vi "writeSVs.vi"(8 "error in (no error)":errorcluster, 11 "LoopTimer in":refnum<class "LoopTimer.lvclass">) -> (0 "error out":errorcluster, 3 "LoopTimer out":refnum<class "LoopTimer.lvclass">)   [LabVIEW 2013, in "ComponentData.lvlib" / "LoopTimer.lvclass"]
uses:
  <userlib>/Common/Component/common_application/RT/ComponentData/LoopTimer/LoopTimer.lvclass
  <userlib>/Common/Component/common_application/RT/ComponentData/LoopTimer/LoopTimer.lvclass/LoopTimer.ctl
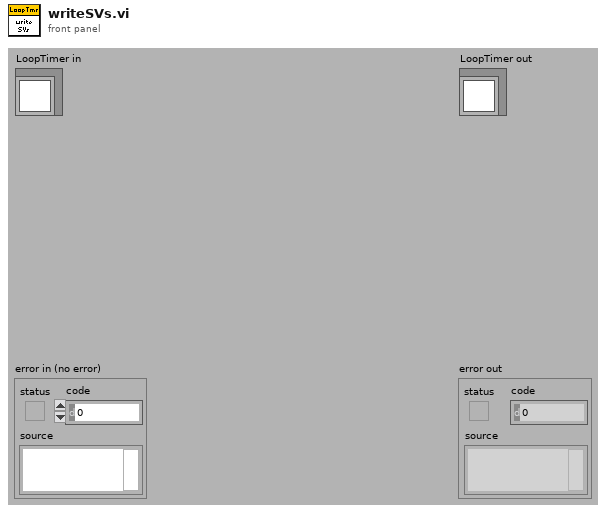
[diagram p1: front panel]
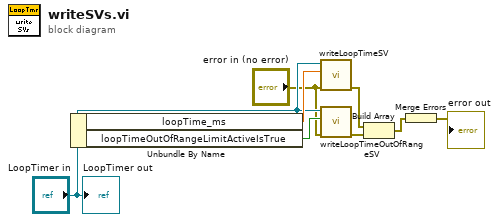
[diagram p0: block diagram]
diagram:
  n1 = Unbundle By Name("LoopTimer in") -> ("loopTime_ms"=w7:dbl, "loopTimeOutOfRangeLimitActiveIsTrue"=w5:bool)
  n2 = call-dynamic "writeLoopTimeSV.vi"("error in (no error)"="error in (no error)", "loopTime_ms"=w7, "LoopTimer in"="LoopTimer in") -> ("error out"=w3:errorcluster)  [unwired: 7 in, 1 out]
  n3 = call-dynamic "writeLoopTimeOutOfRangeSV.vi"("error in (no error)"="error in (no error)", "loopTimeOutOfRangeLimitActiveIsTrue"=w5, "LoopTimer in"="LoopTimer in") -> ("error out"=w2:errorcluster)  [unwired: 7 in, 1 out]
  n4 = Build Array(w3, w2) -> (w1:errorcluster[])
  n5 = Merge Errors(w1) -> (→"error out":errorcluster)
  "LoopTimer out" <- "LoopTimer in"
